vi "Cheesy_Offset.vi"(0 "Communications_Cluster":T1, 2 "Astrom_Cluster":T2 {"GuiderAstrom"."CRVAL" format="%.6g"; "GuiderAstrom"."CD" format="%_7g"; "FieldAstrom"."CRVAL" format="%.6g"; "FieldAstrom"."CD" format="%_7g"; "TablesAstrom"."CRVAL" format="%.6g"; "TablesAstrom"."CD" format="%_7g"}, 5 "RA offset":dbl format="%.2f", 9 "DEC offset":dbl format="%.2f", 11 "VariablesReferences":T3, 13 "OffsetAccuracy (pixels)":dbl=3.0) -> (6 "Error code":u8, 8 "Undo offset":bool, 10 "Warning code":u8, 15 "Error Comment":string)   [LabVIEW 2019]
uses:
  Polymorphics/Distance(single).vi
  Globals.vi
panel:
  in  "MainTAB":enum32{"Entrées", "Locales", "Sories"}(tab)
  in  "USNO_data":string[][](array[string])
  in  "FOV":dbl format="%.2f"
  in  "EPOCH":dbl format="%.2f"
  out "LimXPesto":refnum<vi>
  out "BrasPesto":refnum<vi>
  out "SNR":refnum<vi>
  out "RA before":dbl
  out "DEC before":dbl
  out "StopServo":refnum<vi>
  out "TCS VRN":refnum<visa-resource-name>
  out "Table VRN":refnum<visa-resource-name>
  out "TCS Error":errorcluster
  out "Table Error":errorcluster
  out "FieldAstrom":T4 {"CRVAL" format="%.6g"; "CD" format="%_7g"}
  out "GuiderAstrom":T4 {"CRVAL" format="%.6g"; "CD" format="%_7g"}
  out "TablesAstrom":T4 {"CRVAL" format="%.6g"; "CD" format="%_7g"}
  out "TCS Actif":refnum<vi>
  out "Table Actif":refnum<vi>
  out "StartServo":refnum<vi>
  out "Undo startguide":bool
  out "Guiding":bool caption="Guider was running"
  out "Accesible?":bool
  out "New Source Found ?":bool
  out "RA Moffset":dbl format="%.2f"
  out "DEC Moffset":dbl format="%.2f"
  out "RA Goffset":dbl=10.0 format="%.2f"
  out "DEC Goffset":dbl=10.0 format="%.2f"
  out "Goffset":bool
  out "Moffset":bool
  out "RA after":dbl
  out "DEC after":dbl
  out "cible Y":dbl
  out "cible X":dbl
  out "Servo":refnum<vi>
  out "GuiderMode":u16
  out "Mode":refnum<vi>
  out "FoyerSonde":refnum<vi>
  out "Diff X":refnum<vi>
  out "Diff Y":refnum<vi>
  out "Value X":dbl
  out "Value Y":dbl
  out "TabMove":refnum<vi>
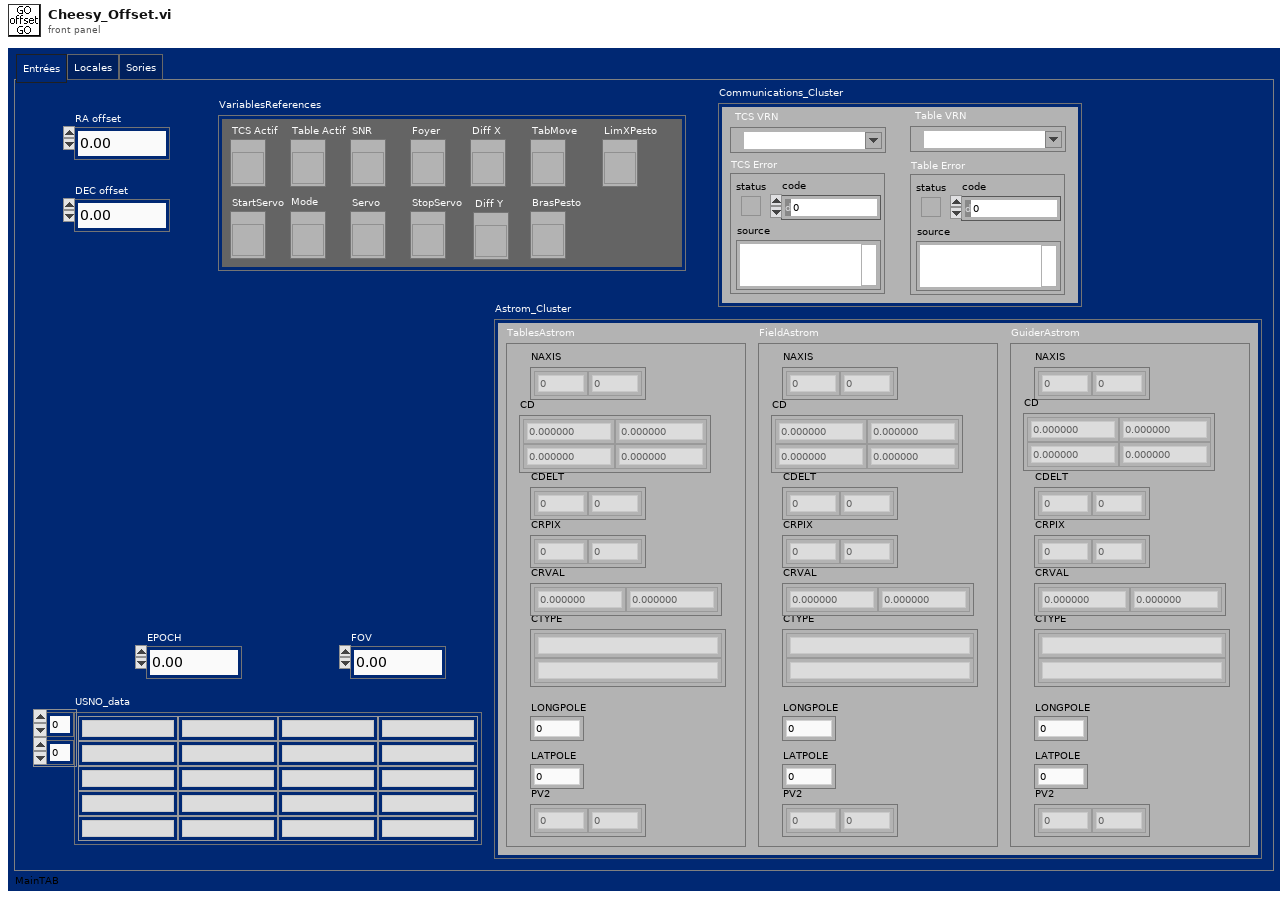
[diagram p1: front panel]
types:
  T1 = cluster{"TCS VRN":refnum<visa-resource-name>, "TCS Error":errorcluster, "Table VRN":refnum<visa-resource-name>, "Table Error":errorcluster}
  T2 = cluster{"TablesAstrom":cluster{"NAXIS":dbl[], "CD":dbl[][], "CDELT":dbl[], "CRPIX":dbl[], "CTYPE":string[], "CRVAL":dbl[], "LONGPOLE":dbl, "LATPOLE":dbl, "PV2":dbl[]}, "FieldAstrom":cluster{"NAXIS":dbl[], "CD":dbl[][], "CDELT":dbl[], "CRPIX":dbl[], "CTYPE":string[], "CRVAL":dbl[], "LONGPOLE":dbl, "LATPOLE":dbl, "PV2":dbl[]}, "GuiderAstrom":cluster{"NAXIS":dbl[], "CD":dbl[][], "CDELT":dbl[], "CRPIX":dbl[], "CTYPE":string[], "CRVAL":dbl[], "LONGPOLE":dbl, "LATPOLE":dbl, "PV2":dbl[]}}
  T3 = cluster{"TCS Actif":refnum<vi>, "Table Actif":refnum<vi>, "Foyer":refnum<vi>, "StartServo":refnum<vi>, "Mode":refnum<vi>, "Servo":refnum<vi>, "StopServo":refnum<vi>, "Diff X":refnum<vi>, "Diff Y":refnum<vi>, "SNR":refnum<vi>, "TabMove":refnum<vi>, "BrasPesto":refnum<vi>, "LimXPesto":refnum<vi>}
  T4 = cluster{"NAXIS":dbl[], "CD":dbl[][], "CDELT":dbl[], "CRPIX":dbl[], "CTYPE":string[], "CRVAL":dbl[], "LONGPOLE":dbl, "LATPOLE":dbl, "PV2":dbl[]}
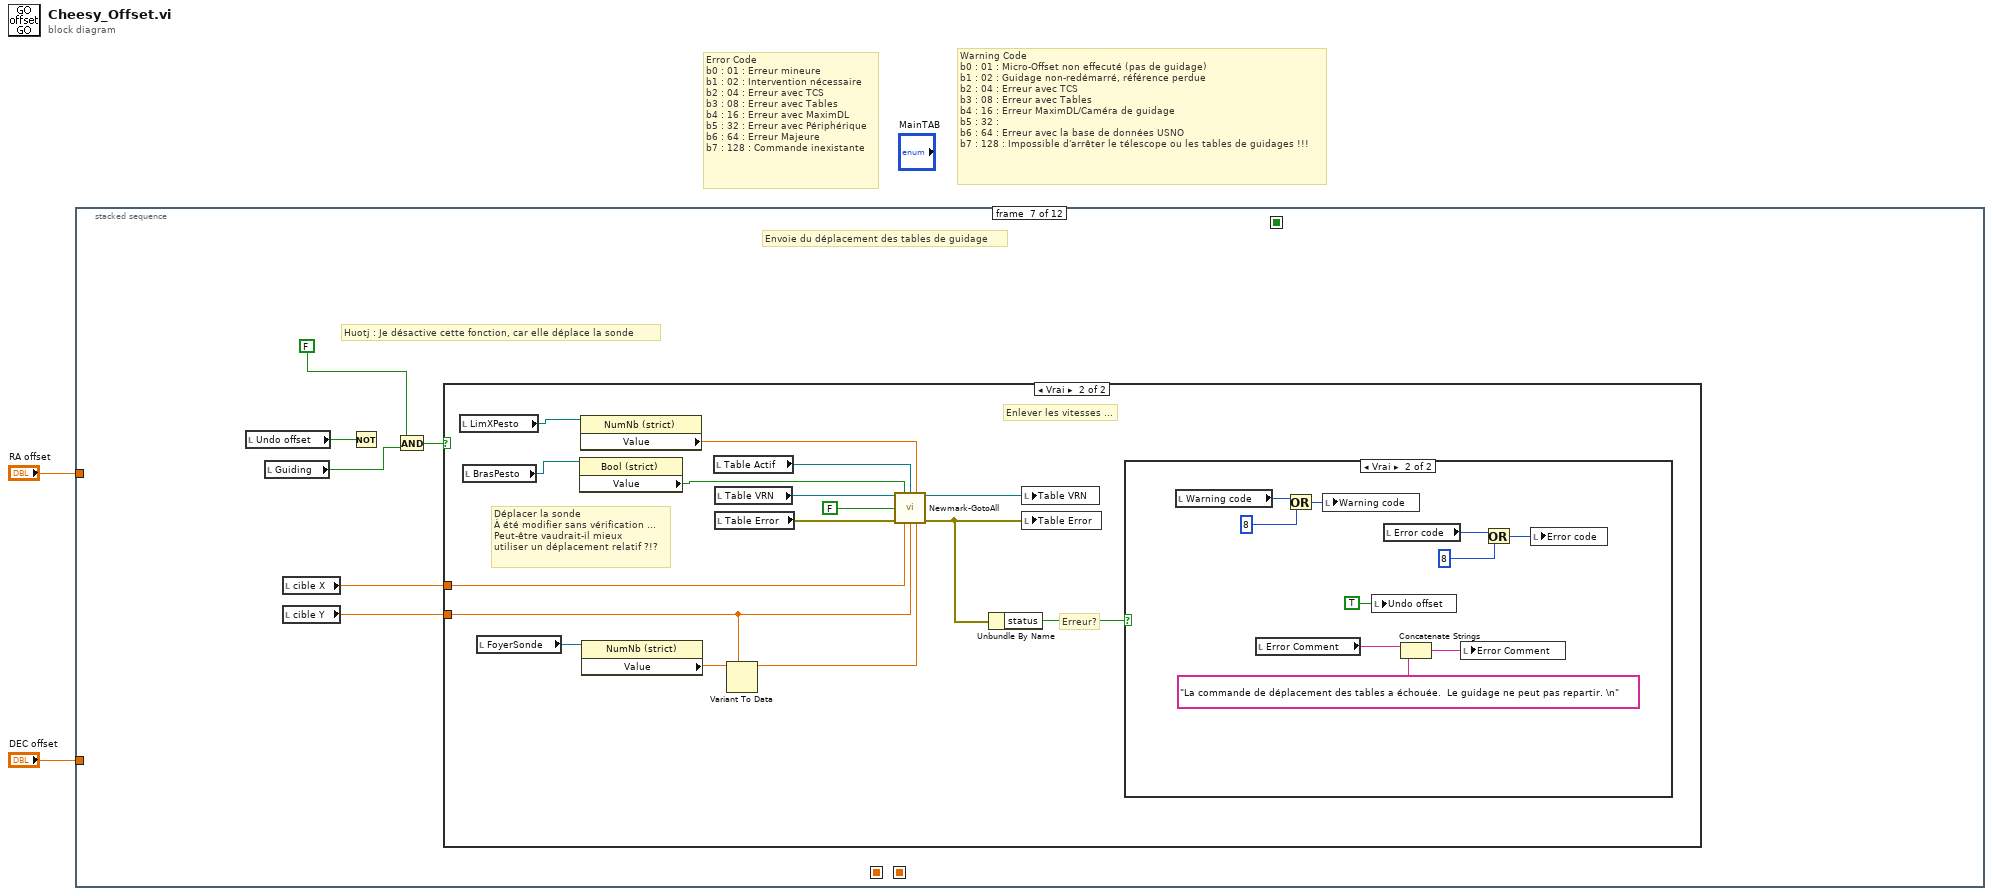
[diagram p0: block diagram]
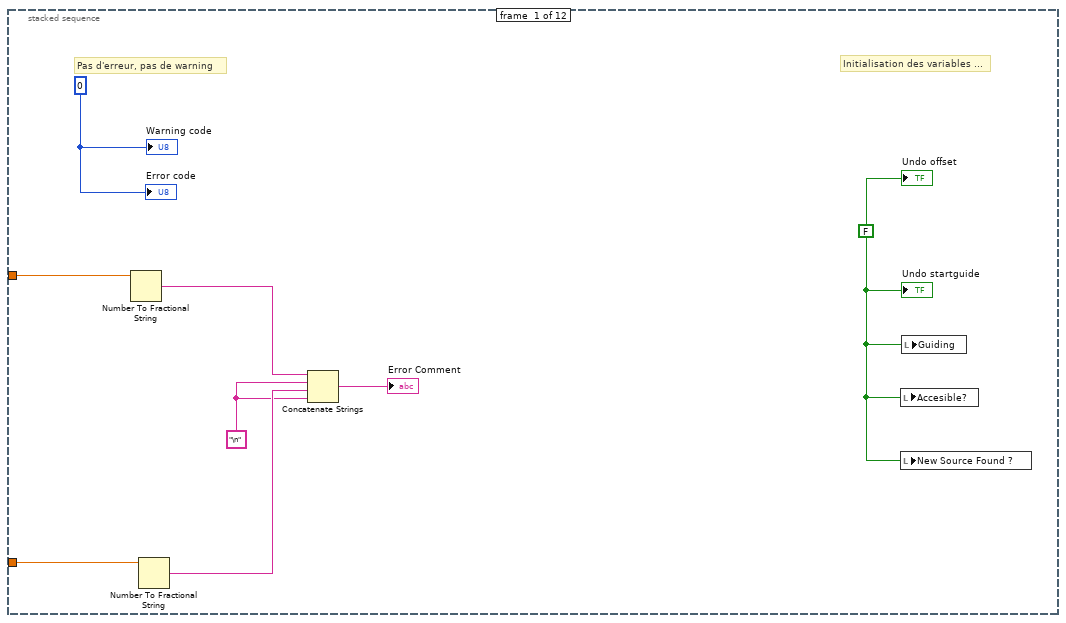
[diagram p2: hidden frame]
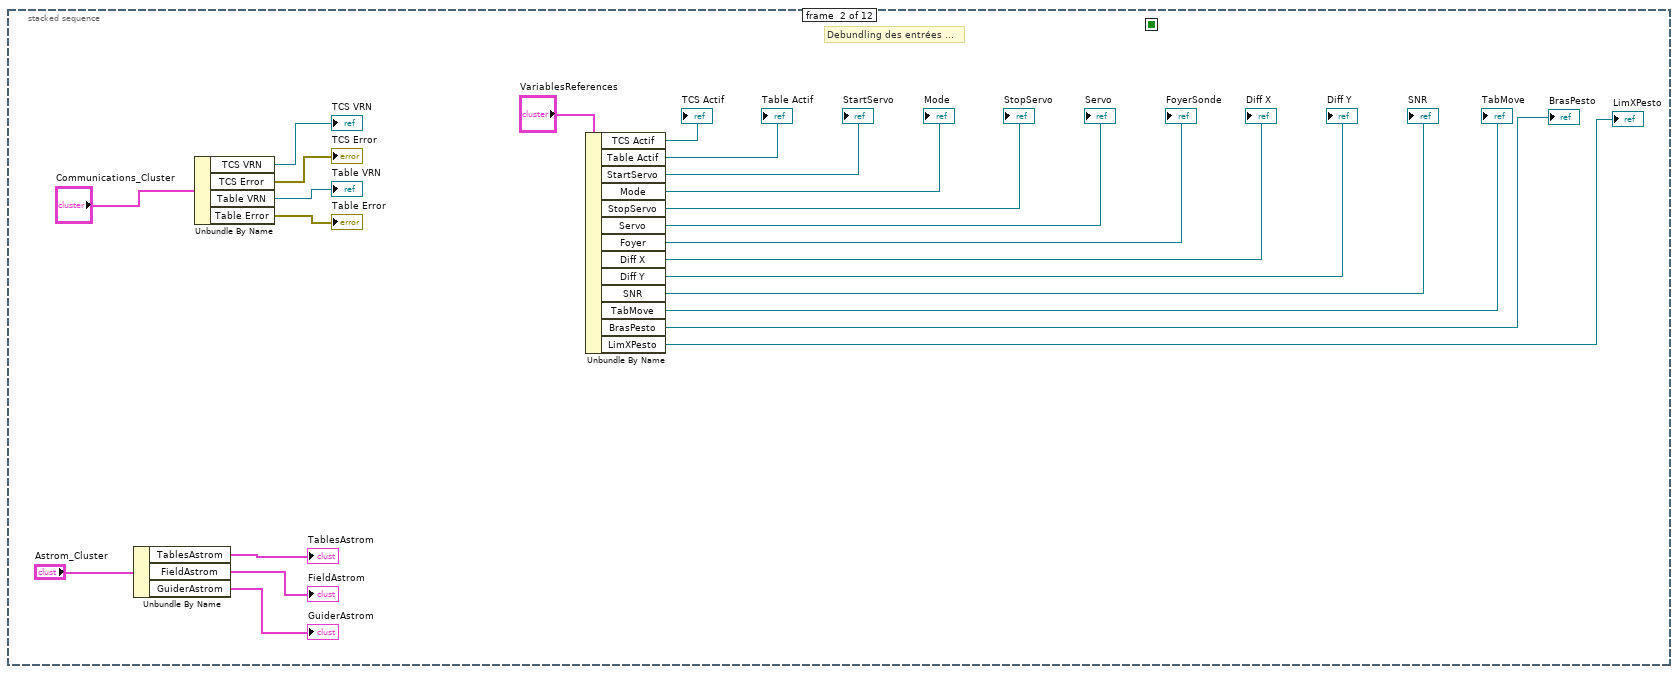
[diagram p3: hidden frame]
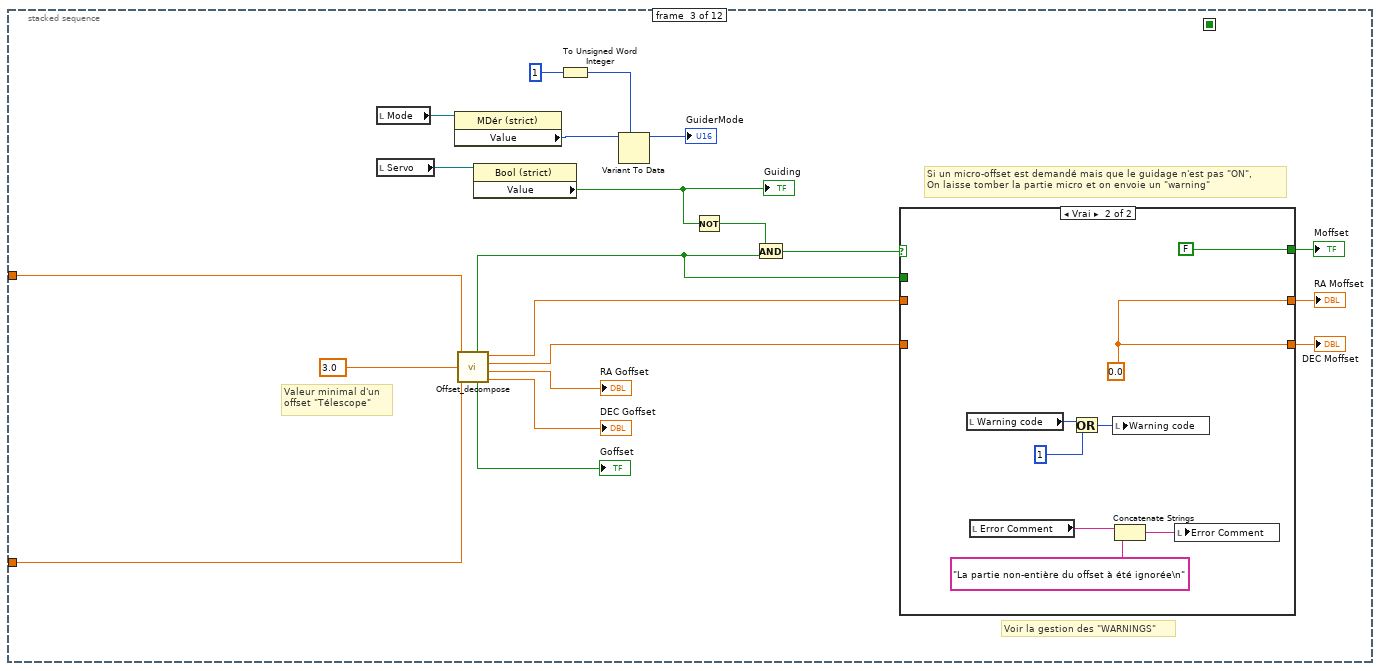
[diagram p4: hidden frame]
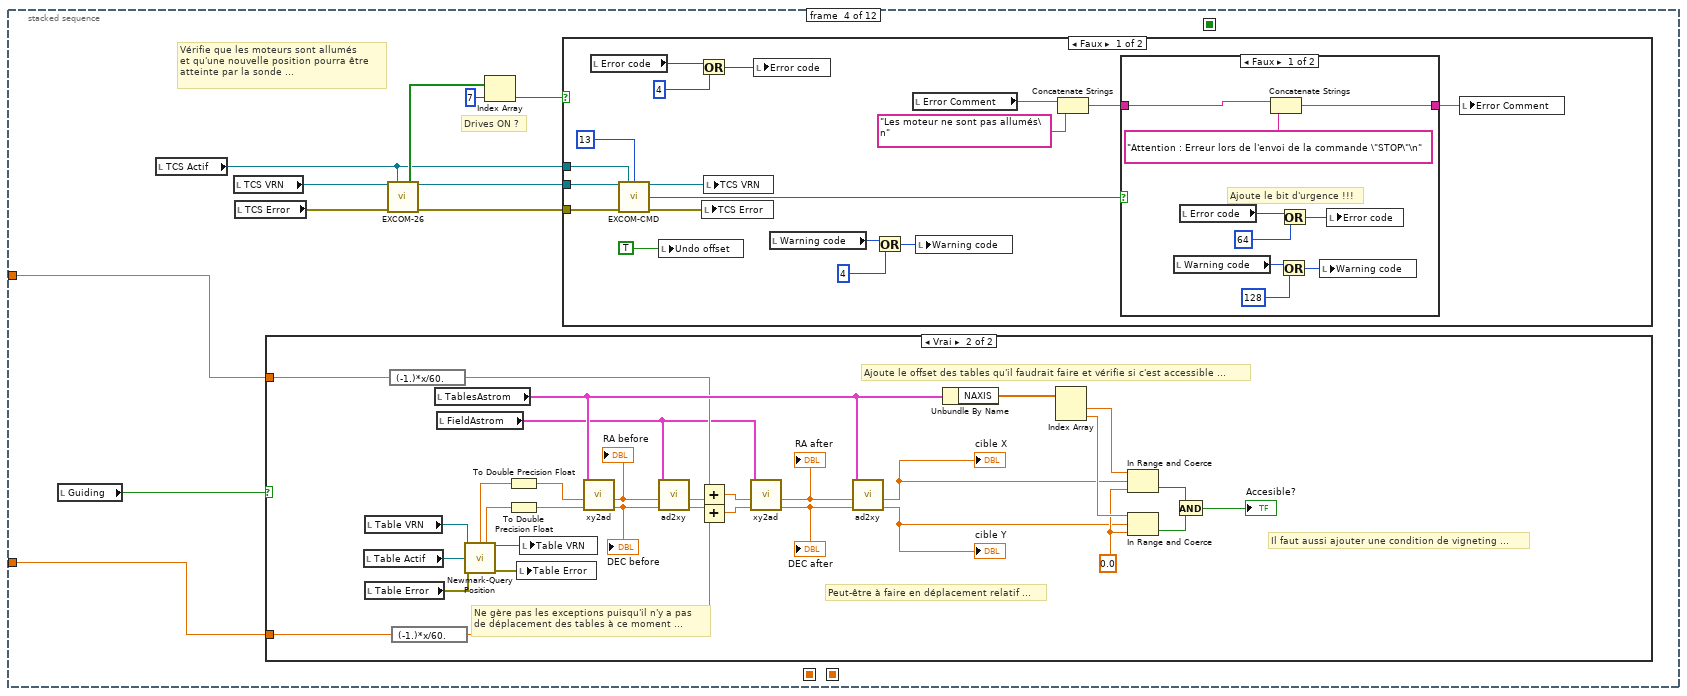
[diagram p6: hidden frame]
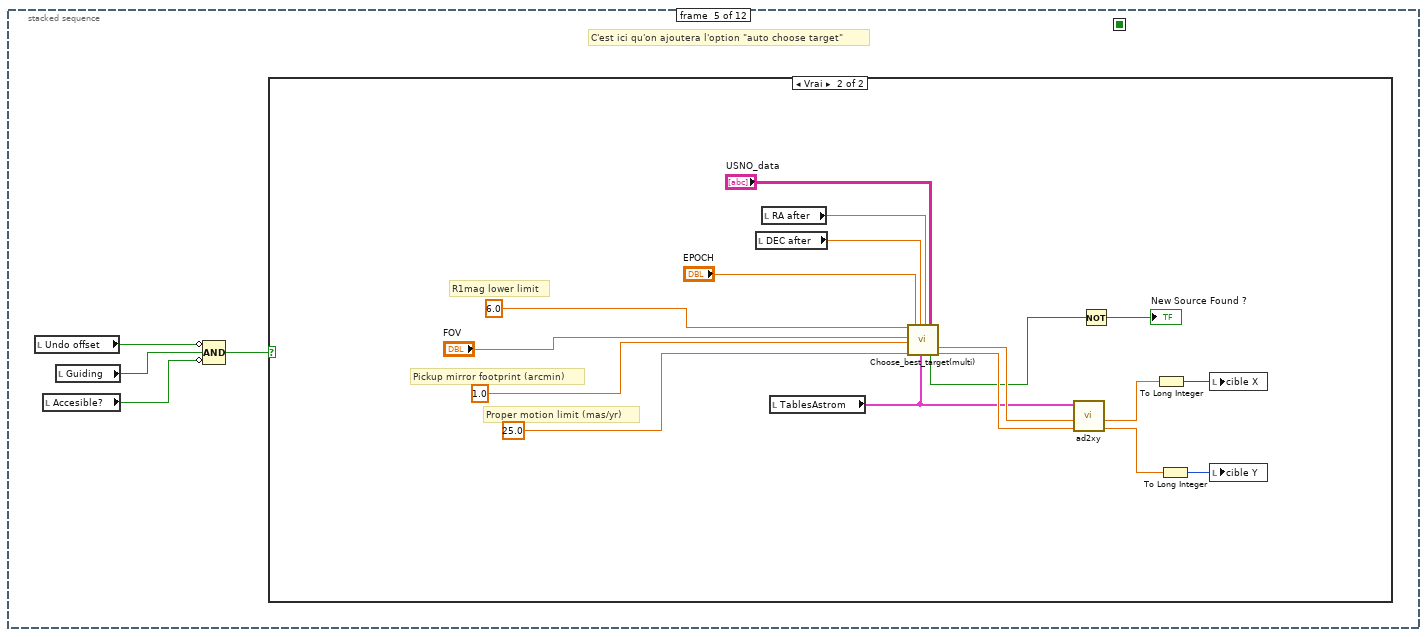
[diagram p10: hidden frame]
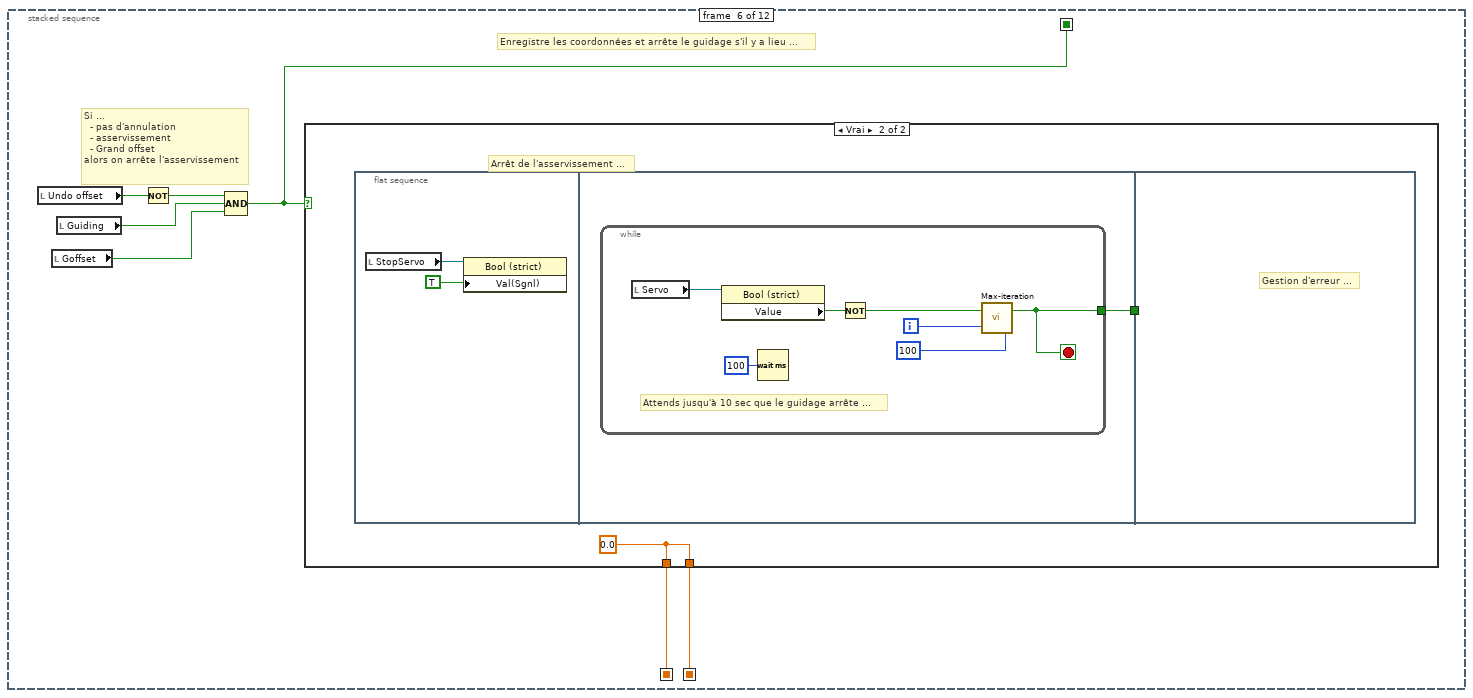
[diagram p12: hidden frame]
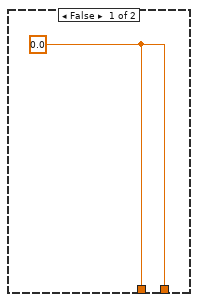
[diagram p13: hidden frame]
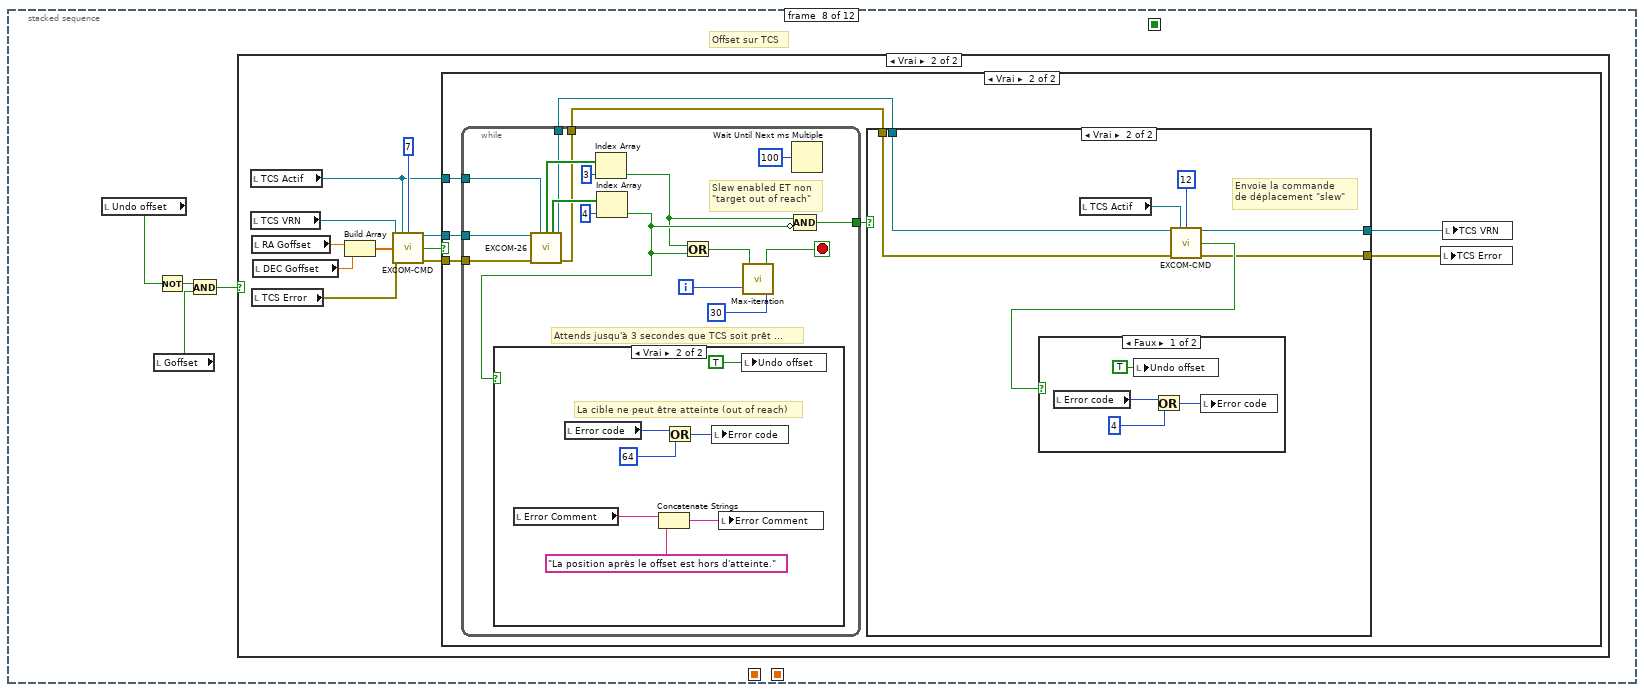
[diagram p16: hidden frame]
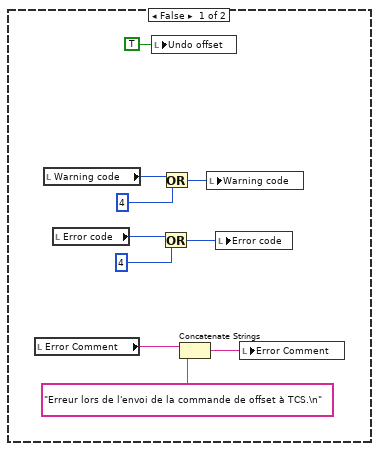
[diagram p18: hidden frame]
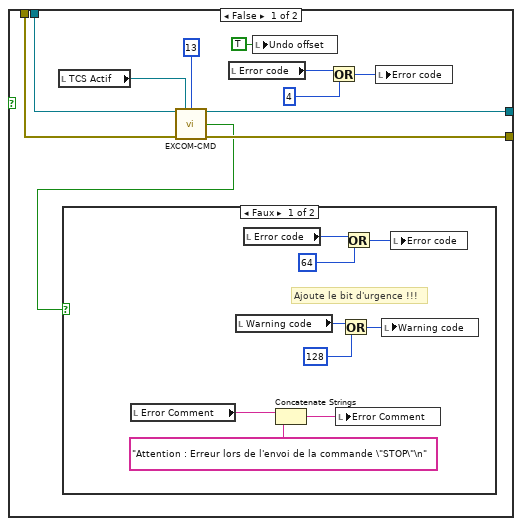
[diagram p20: hidden frame]
diagram:
  # "Error Code\nb0 : 01 : Erreur mineure\nb1 : 02 : Intervention nécessaire\nb2 : 04 : Erreur avec TCS\nb3 : 08 : Erreur avec Tables\nb4 : 16 : Erreur avec MaximDL\nb5 : 32 : Erreur avec Périphérique\nb6 : 64 : Erreur Majeure\nb7 : 128 : Commande inexistante"
  # "Warning Code\nb0 : 01 : Micro-Offset non effecuté (pas de guidage)\nb1 : 02 : Guidage non-redémarré, référence perdue\nb2 : 04 : Erreur avec TCS\nb3 : 08 : Erreur avec Tables\nb4 : 16 : Erreur MaximDL/Caméra de guidage\nb5 : 32 : \nb6 : 64 : Erreur avec la base de données USNO\nb7 : 128 : Impossible d'arrêter le télescope ou les tables de guidages !!!"
  n1 = stacked-sequence {
    seq-local: [_ _ _ _ _ w161 _ _ _ _ _ _] -> [_ _ _ _ _ _ _ _ _ _ _ _]
    seq-local: [_ _ _ _ _ w160 _ _ _ _ _ _] -> [_ _ _ _ _ _ _ _ _ _ _ _]
    seq-local: [_ _ _ _ _ w159 _ _ _ _ _ _] -> [_ _ _ _ _ _ _ _ _ _ _ _]
    tunnel: "DEC offset" -> [w7 _ w53 w74 _ _ _ _ _ _ _ _]
    tunnel: "RA offset" -> [w8 _ w54 w73 _ _ _ _ _ _ _ _]
    frame #0 {
      w3 = "\n"
      w9 = FALSE
      w10 = u8 0
      # "Initialisation des variables ..."
      # "Pas d'erreur, pas de warning"
      n2 = Number To Fractional String(number=w8) -> (F-format string=w6:string)  [unwired: 3 in]
      n3 = Number To Fractional String(number=w7) -> (F-format string=w5:string)  [unwired: 3 in]
      n4 = Concatenate Strings(w6, w3, w5, w3) -> (→"Error Comment":string)
      n5 = local write "Accesible?"(w9) -> ()
      n6 = local write "New Source Found ?"(w9) -> ()
      n7 = local write "Guiding"(w9) -> ()
      "Error code" <- w10
      "Warning code" <- w10
      "Undo offset" <- w9
      "Undo startguide" <- w9
    }
    frame #1 {
      # "Debundling des entrées ..."
      n8 = Unbundle By Name("Astrom_Cluster") -> ("TablesAstrom"=→"TablesAstrom":T4, "FieldAstrom"=→"FieldAstrom":T4, "GuiderAstrom"=→"GuiderAstrom":T4)
      n9 = Unbundle By Name("Communications_Cluster") -> ("TCS VRN"=→"TCS VRN":refnum<visa-resource-name>, "TCS Error"=→"TCS Error":errorcluster, "Table VRN"=→"Table VRN":refnum<visa-resource-name>, "Table Error"=→"Table Error":errorcluster)
      n10 = Unbundle By Name("VariablesReferences") -> ("TCS Actif"=→"TCS Actif":refnum<vi>, "Table Actif"=→"Table Actif":refnum<vi>, "StartServo"=→"StartServo":refnum<vi>, "Mode"=→"Mode":refnum<vi>, "StopServo"=→"StopServo":refnum<vi>, "Servo"=→"Servo":refnum<vi>, "Foyer"=→"FoyerSonde":refnum<vi>, "Diff X"=→"Diff X":refnum<vi>, "Diff Y"=→"Diff Y":refnum<vi>, "SNR"=→"SNR":refnum<vi>, "TabMove"=→"TabMove":refnum<vi>, "BrasPesto"=→"BrasPesto":refnum<vi>, "LimXPesto"=→"LimXPesto":refnum<vi>)
    }
    frame #2 {
      # "Voir la gestion des \"WARNINGS\""
      # "Si un micro-offset est demandé mais que le guidage n'est pas \"ON\",\nOn laisse tomber la partie micro et on envoie un \"warning\""
      # "Valeur minimal d'un\noffset \"Télescope\""
      n11 = local read "Mode"() -> (w34:refnum<vi>)
      n12 = local read "Servo"() -> (w40:refnum<vi>)
      n13 = property class="MDér (strict)"(reference=w34) -> ("Value"=w38:u16)  [unwired: 1 in, 2 out]
      n14 = call "Offset_decompose.vi"("DEC offset"=w53, "RA offset"=w54, "Micro Limit"=3.0 ("y")) -> ("Goffset"=→"Goffset":bool, "Moffset"=w43:bool, "DEC Goffset"=→"DEC Goffset":dbl, "RA Goffset"=→"RA Goffset":dbl, "DEC Moffset"=w47:dbl, "RA Moffset"=w48:dbl)  [unwired: 2 in]
      n15 = property class="Bool (strict)"(reference=w40) -> ("Value"=w39:bool)  [unwired: 1 in, 2 out]
      "Guiding" <- w39
      n16 = To Unsigned Word Integer(number=u8 1) -> (unsigned 16bit integer=w36:u16)
      n17 = Variant To Data(type=w36, Variant=w38) -> (data=→"GuiderMode":u16)  [unwired: 1 in, 1 out]
      n18 = Not(x=w39) -> (.not. x?=w49:bool)
      n19 = And(x=w49, y=w43) -> (x .and. y?=w44:bool)
      n20 = case shown="Vrai" w44 {
        tunnel: w48 -> [w57 _]
        tunnel: w47 -> [w56 _]
        tunnel: [w57 w64] -> w46
        tunnel: [w56 w64] -> w45
        tunnel: w43 -> [w55 _]
        tunnel: [w55 FALSE] -> w41
        frame False {
        }
        frame True {
          w64 = 0.0
          n21 = local read "Warning code"() -> (w63:u8)
          n22 = local read "Error Comment"() -> (w60:string)
          n23 = Or(x=w63, y=u8 1) -> (x .or. y?=w62:u8)
          n24 = local write "Warning code"(w62) -> ()
          n25 = Concatenate Strings(w60, "La partie non-entière du offset à été ignorée\n") -> (w59:string)
          n26 = local write "Error Comment"(w59) -> ()
        }
      }
      "DEC Moffset" <- w45
      "RA Moffset" <- w46
      "Moffset" <- w41
    }
    frame #3 {
      # "Drives ON ?"
      # "Vérifie que les moteurs sont allumés\net qu'une nouvelle position pourra être\natteinte par la sonde ..."
      n27 = local read "Guiding"() -> (w72:bool)
      n28 = local read "TCS Actif"() -> (w68:refnum<vi>)
      n29 = local read "TCS VRN"() -> (w67:refnum<visa-resource-name>)
      n30 = local read "TCS Error"() -> (w66:errorcluster)
      n31 = case shown="Vrai" w72 {
        tunnel: w74 -> [_ w106]
        tunnel: w73 -> [_ w105]
        frame False {
        }
        frame True {
          w98 = 0.0
          # "Peut-être à faire en déplacement relatif ..."
          # "Ne gère pas les exceptions puisqu'il n'y a pas\nde déplacement des tables à ce moment ..."
          # "Il faut aussi ajouter une condition de vigneting ..."
          # "Ajoute le offset des tables qu'il faudrait faire et vérifie si c'est accessible ..."
          n32 = local read "Table Actif"() -> (w84:refnum<vi>)
          n33 = local read "Table VRN"() -> (w82:refnum<visa-resource-name>)
          n34 = local read "Table Error"() -> (w80:errorcluster)
          n35 = expression code="(-1.)*x/60."(w105) -> (w94:dbl)
          n36 = expression code="(-1.)*x/60."(w106) -> (w93:dbl)
          n37 = local read "TablesAstrom"() -> (w104:T4)
          n38 = local read "FieldAstrom"() -> (w83:T4)
          n39 = call "Newmark-QueryPosition.vi"("Table VRN IN"=w82, "Bool Refnum"=w84, "Error IN"=w80) -> ("X Axis"=w86:dbl, "Y Axis"=w85:dbl, "Table VRN OUT"=w79:refnum<visa-resource-name>, "Error OUT"=w81:errorcluster)  [unwired: 5 in, 4 out]
          n40 = To Double Precision Float(number=w86) -> (double precision float=w108:dbl)
          n41 = To Double Precision Float(number=w85) -> (double precision float=w107:dbl)
          n42 = local write "Table Error"(w81) -> ()
          n43 = local write "Table VRN"(w79) -> ()
          n44 = call "xy2ad.vi"("Y (px)"=w107, "X (px)"=w108, "Astrometry"=w104) -> ("DEC (°)"=w77:dbl, "RA (°)"=w78:dbl)  [unwired: 5 in, 2 out]
          "RA before" <- w78
          "DEC before" <- w77
          n45 = call "ad2xy.vi"("DEC"=w77, "RA"=w78, "Astrometry"=w83) -> ("Y"=w95:dbl, "X"=w96:dbl)  [unwired: 6 in, 1 out]
          n46 = Add(x=w94, y=w96) -> (x+y=w92:dbl)
          n47 = Add(x=w95, y=w93) -> (x+y=w91:dbl)
          n48 = call "xy2ad.vi"("Y (px)"=w91, "X (px)"=w92, "Astrometry"=w83) -> ("DEC (°)"=w89:dbl, "RA (°)"=w90:dbl)  [unwired: 5 in, 2 out]
          "DEC after" <- w89
          "RA after" <- w90
          n49 = call "ad2xy.vi"("DEC"=w89, "RA"=w90, "Astrometry"=w104) -> ("Y"=w87:dbl, "X"=w88:dbl)  [unwired: 6 in, 1 out]
          "cible X" <- w88
          "cible Y" <- w87
          n50 = Unbundle By Name(w104) -> ("NAXIS"=w103:dbl[])
          n51 = Index Array(array=w103) -> (element #1=w102:dbl, element #2=w101:dbl)  [unwired: 2 in]
          n52 = In Range and Coerce(upper limit=w102, x=w88, lower limit=w98) -> (In Range?=w100:bool)  [unwired: 1 out]
          n53 = In Range and Coerce(upper limit=w101, x=w87, lower limit=w98) -> (In Range?=w99:bool)  [unwired: 1 out]
          n54 = And(x=w100, y=w99) -> (x .and. y?=→"Accesible?":bool)
        }
      }
      n55 = call "EXCOM-26.vi"("VRN IN"=w67, "Bool Refnum"=w68, "Error IN"=w66) -> ("STATH"=w70:bool[], "VRN OUT"=w75:refnum<visa-resource-name>, "Error OUT"=w69:errorcluster)  [unwired: 6 in, 4 out]
      n56 = Index Array(array=w70, index=7 ("Index")) -> (element=w76:bool)
      n57 = case shown="Faux" w76 {
        tunnel: w75 -> [w121 _]
        tunnel: w69 -> [w116 _]
        tunnel: w68 -> [w115 _]
        frame False {
          n58 = local read "Error code"() -> (w126:u8)
          n59 = call "EXCOM-CMD.vi"("VRN IN"=w121, "Bool Refnum"=w115, "Commande #"=13 ("NombredArguments"), "Error IN"=w116) -> ("VRN OUT"=w110:refnum<visa-resource-name>, "OK Done"=w122:bool, "Error OUT"=w109:errorcluster)  [unwired: 9 in]
          n60 = local write "Undo offset"(TRUE) -> ()
          n61 = Or(x=w126, y=u8 4) -> (x .or. y?=w125:u8)
          n62 = local write "TCS Error"(w109) -> ()
          n63 = local write "TCS VRN"(w110) -> ()
          n64 = local write "Error code"(w125) -> ()
          n65 = local read "Warning code"() -> (w120:u8)
          n66 = Or(x=w120, y=u8 4) -> (x .or. y?=w119:u8)
          n67 = local read "Error Comment"() -> (w114:string)
          n68 = local write "Warning code"(w119) -> ()
          n69 = Concatenate Strings(w114, "Les moteur ne sont pas allumés\n") -> (w112:string)
          n70 = case shown="Faux" w122 {
            tunnel: w112 -> [w129 w136]
            tunnel: [w128 w136] -> w111
            frame False {
              # "Ajoute le bit d'urgence !!!"
              n71 = local read "Warning code"() -> (w133:u8)
              n72 = local read "Error code"() -> (w132:u8)
              n73 = Concatenate Strings(w129, "Attention : Erreur lors de l'envoi de la commande \"STOP\"\n" ("string")) -> (w128:string)
              n74 = Or(x=w133, y=u8 128) -> (x .or. y?=w134:u8)
              n75 = Or(x=w132, y=u8 64) -> (x .or. y?=w131:u8)
              n76 = local write "Warning code"(w134) -> ()
              n77 = local write "Error code"(w131) -> ()
            }
            frame True {
            }
          }
          n78 = local write "Error Comment"(w111) -> ()
        }
        frame True {
        }
      }
    }
    frame #4 {
      # "C'est ici qu'on ajoutera l'option \"auto choose target\""
      n79 = local read "Undo offset"() -> (w140:bool)
      n80 = local read "Accesible?"() -> (w138:bool)
      n81 = local read "Guiding"() -> (w139:bool)
      n82 = Compound Arithmetic op=AND(invert w140, w139, invert w138) -> (w137:bool)
      n83 = case shown="Vrai" w137 {
        frame False {
        }
        frame True {
          # "Proper motion limit (mas/yr)"
          # "Pickup mirror footprint (arcmin)"
          # "R1mag lower limit"
          n84 = local read "DEC after"() -> (w156:dbl)
          n85 = local read "RA after"() -> (w157:dbl)
          n86 = local read "TablesAstrom"() -> (w147:T4)
          n87 = call "Choose_best_target(multi).vi"("R1mag lower limit"=6.0, "FOV"="FOV", "Footprint"=1.0, "PM limit"=25.0 ("Footprint"), "EPOCH TEL"="EPOCH", "DEC TEL"=w156, "Table Astrometry"=w147, "RA TEL"=w157, "USNO_data"="USNO_data") -> ("erreur"=w142:bool, "target RA (deg)"=w150:dbl, "target DEC (deg)"=w149:dbl)  [unwired: 3 in, 5 out]
          n88 = call "ad2xy.vi"("DEC"=w149, "RA"=w150, "Astrometry"=w147) -> ("Y"=w151:dbl, "X"=w152:dbl)  [unwired: 6 in, 1 out]
          n89 = Not(x=w142) -> (.not. x?=→"New Source Found ?":bool)
          n90 = To Long Integer(number=w152) -> (32bit integer=w154:i32)
          n91 = To Long Integer(number=w151) -> (32bit integer=w153:i32)
          n92 = local write "cible X"(w154) -> ()
          n93 = local write "cible Y"(w153) -> ()
        }
      }
    }
    frame #5 {
      # "Si ...\n  - pas d'annulation\n  - asservissement\n  - Grand offset\nalors on arrête l'asservissement"
      # "Enregistre les coordonnées et arrête le guidage s'il y a lieu ..."
      n94 = local read "Undo offset"() -> (w163:bool)
      n95 = local read "Goffset"() -> (w158:bool)
      n96 = local read "Guiding"() -> (w162:bool)
      n97 = Not(x=w163) -> (.not. x?=w164:bool)
      n98 = Compound Arithmetic op=AND(w164, w162, w158) -> (w161:bool)
      n99 = case shown="Vrai" w161 {
        tunnel: [w165 w167] -> w159
        tunnel: [w165 w167] -> w160
        frame False {
          w165 = sgl 0.0 ("GuiderYError")
        }
        frame True {
          w167 = sgl 0.0 ("GuiderYError")
          # "Arrêt de l'asservissement ..."
          n100 = flat-sequence {
            tunnel: [w170] -> w166
            tunnel: w166 -> [_]
            frame #0 {
              n101 = local read "StopServo"() -> (w169:refnum<vi>)
              n102 = property class="Bool (strict)"(reference=w169, "Val(Sgnl)"=TRUE ("Value (Signaling)")) -> ()  [unwired: 1 in, 2 out]
            }
            frame #1 {
              n103 = while {
                tunnel: [w172] -> w170
                i -> [w175]
                stop <- w172 stop-if-true
                # "Attends jusqu'à 10 sec que le guidage arrête ..."
                n104 = local read "Servo"() -> (w177:refnum<vi>)
                n105 = property class="Bool (strict)"(reference=w177) -> ("Value"=w176:bool)  [unwired: 1 in, 2 out]
                n106 = Wait (ms)(milliseconds to wait=u32 100) -> ()  [unwired: 1 out]
                n107 = Not(x=w176) -> (.not. x?=w171:bool)
                n108 = call "Max-iteration.vi"("i max"=100, "i act"=w175, "Valeur entrante"=w171) -> ("break ?"=w172:bool)
              }
            }
            frame #2 {
              # "Gestion d'erreur ..."
            }
          }
        }
      }
    }
    frame #6 {
      # "Huotj : Je désactive cette fonction, car elle déplace la sonde"
      # "Envoie du déplacement des tables de guidage"
      n109 = local read "Undo offset"() -> (w180:bool)
      n110 = local read "Guiding"() -> (w179:bool)
      n111 = local read "cible X"() -> (w183:dbl)
      n112 = local read "cible Y"() -> (w182:dbl)
      n113 = Not(x=w180) -> ()  [unwired: 1 out]
      n114 = And(x=FALSE, y=w179) -> (x .and. y?=w181:bool)
      n115 = case shown="Vrai" w181 {
        tunnel: w182 -> [_ w189]
        tunnel: w183 -> [_ w198]
        frame False {
        }
        frame True {
          # "Erreur?"
          # "Enlever les vitesses ..."
          # "Déplacer la sonde\nÀ été modifier sans vérification ...\nPeut-être vaudrait-il mieux\nutiliser un déplacement relatif ?!?"
          n116 = local read "LimXPesto"() -> (w187:refnum<vi>)
          n117 = local read "BrasPesto"() -> (w185:refnum<vi>)
          n118 = local read "FoyerSonde"() -> (w191:refnum<vi>)
          n119 = property class="Bool (strict)"(reference=w185) -> ("Value"=w184:bool)  [unwired: 1 in, 2 out]
          n120 = property on="Property Node" class="NumNb (strict)"(reference=w187) -> ("Value"=w186:dbl)  [unwired: 1 in, 2 out]
          n121 = property on="Property Node" class="NumNb (strict)"(reference=w191) -> ("Value"=w190:dbl)  [unwired: 1 in, 2 out]
          n122 = local read "Table Actif"() -> (w195:refnum<vi>)
          n123 = local read "Table VRN"() -> (w193:refnum<visa-resource-name>)
          n124 = local read "Table Error"() -> (w194:errorcluster)
          n125 = Variant To Data(type=w189, Variant=w190) -> (data=w188:dbl)  [unwired: 1 in, 1 out]
          n126 = call "Newmark-GotoAll.vi"("Table VRN IN"=w193, "BrasPesto"=w184, "Bool Refnum"=w195, "LimXPesto"=w186, "Notify?"=FALSE, "Error IN"=w194, "Position X"=w198, "Position Y"=w189, "Position Z"=w188) -> ("Table VRN OUT"=w196:refnum<visa-resource-name>, "Error OUT"=w197:errorcluster)  [unwired: 5 in]
          n127 = Unbundle By Name(w197) -> ("status"=w199:bool)
          n128 = local write "Table VRN"(w196) -> ()
          n129 = local write "Table Error"(w197) -> ()
          n130 = case shown="Vrai" w199 {
            frame False {
            }
            frame True {
              n131 = local read "Warning code"() -> (w205:u8)
              n132 = local read "Error Comment"() -> (w202:string)
              n133 = Or(x=w205, y=u8 8) -> (x .or. y?=w204:u8)
              n134 = local write "Warning code"(w204) -> ()
              n135 = local write "Undo offset"(TRUE) -> ()
              n136 = local read "Error code"() -> (w206:u8)
              n137 = Concatenate Strings(w202, "La commande de déplacement des tables a échouée.  Le guidage ne peut pas repartir. \n") -> (w201:string)
              n138 = local write "Error Comment"(w201) -> ()
              n139 = Or(x=w206, y=u8 8) -> (x .or. y?=w207:u8)
              n140 = local write "Error code"(w207) -> ()
            }
          }
        }
      }
    }
    frame #7 {
      # "Offset sur TCS"
      n141 = local read "Undo offset"() -> (w211:bool)
      n142 = local read "Goffset"() -> (w210:bool)
      n143 = Not(x=w211) -> (.not. x?=w212:bool)
      n144 = And(x=w212, y=w210) -> (x .and. y?=w213:bool)
      n145 = case shown="Vrai" w213 {
        frame False {
        }
        frame True {
          n146 = local read "TCS Actif"() -> (w216:refnum<vi>)
          n147 = local read "TCS VRN"() -> (w214:refnum<visa-resource-name>)
          n148 = local read "RA Goffset"() -> (w218:dbl)
          n149 = local read "TCS Error"() -> (w215:errorcluster)
          n150 = local read "DEC Goffset"() -> (w219:dbl)
          n151 = Build Array(w218, w219) -> (w217:dbl[])
          n152 = call "EXCOM-CMD.vi"("VRN IN"=w214, "Bool Refnum"=w216, "Commande #"=7 ("NombredArguments"), "Args"=w217, "Error IN"=w215) -> ("VRN OUT"=w222:refnum<visa-resource-name>, "OK Done"=w223:bool, "Error OUT"=w220:errorcluster)  [unwired: 8 in]
          n153 = case shown="Vrai" w223 {
            tunnel: w222 -> [_ w240]
            tunnel: w220 -> [_ w238]
            tunnel: w216 -> [_ w236]
            frame False {
              n154 = local read "Error Comment"() -> (w226:string)
              n155 = local read "Warning code"() -> (w227:u8)
              n156 = local read "Error code"() -> (w232:u8)
              n157 = local write "Undo offset"(TRUE) -> ()
              n158 = Or(x=w232, y=u8 4) -> (x .or. y?=w231:u8)
              n159 = Or(x=w227, y=u8 4) -> (x .or. y?=w228:u8)
              n160 = Concatenate Strings(w226, "Erreur lors de l'envoi de la commande de offset à TCS.\n") -> (w225:string)
              n161 = local write "Warning code"(w228) -> ()
              n162 = local write "Error code"(w231) -> ()
              n163 = local write "Error Comment"(w225) -> ()
            }
            frame True {
              n164 = while {
                tunnel: [w245] -> w241
                tunnel: w240 -> [w253]
                tunnel: [w252] -> w239
                tunnel: w238 -> [w244]
                tunnel: [w243] -> w237
                tunnel: w236 -> [w242]
                i -> [w249]
                stop <- w250 stop-if-true
                # "Slew enabled ET non\n\"target out of reach\""
                # "Attends jusqu'à 3 secondes que TCS soit prêt ..."
                n165 = call "EXCOM-26.vi"("VRN IN"=w253, "Bool Refnum"=w242, "Error IN"=w244) -> ("STATL"=w255:bool[], "STATH"=w254:bool[], "VRN OUT"=w252:refnum<visa-resource-name>, "Error OUT"=w243:errorcluster)  [unwired: 6 in, 3 out]
                n166 = Index Array(array=w255, index=3 ("Index")) -> (element=w246:bool)
                n167 = Index Array(array=w254, index=4 ("Index")) -> (element=w247:bool)
                n168 = case shown="Vrai" w247 {
                  frame False {
                  }
                  frame True {
                    # "La cible ne peut être atteinte (out of reach)"
                    n169 = local read "Error Comment"() -> (w261:string)
                    n170 = local read "Error code"() -> (w265:u8)
                    n171 = Concatenate Strings(w261, "La position après le offset est hors d'atteinte.") -> (w260:string)
                    n172 = Or(x=w265, y=u8 64) -> (x .or. y?=w264:u8)
                    n173 = local write "Error code"(w264) -> ()
                    n174 = local write "Error Comment"(w260) -> ()
                    n175 = local write "Undo offset"(TRUE ("Undo offset")) -> ()
                  }
                }
                n176 = Or(x=w246, y=w247) -> (x .or. y?=w251:bool)
                n177 = call "Max-iteration.vi"("i max"=30, "i act"=w249, "Valeur entrante"=w251) -> ("break ?"=w250:bool)
                n178 = Wait Until Next ms Multiple(millisecond multiple=u32 100 ("n millisecondes")) -> ()  [unwired: 1 out]
                n179 = Compound Arithmetic op=AND(w246, invert w247) -> (w245:bool)
              }
              n180 = case shown="Vrai" w241 {
                tunnel: w239 -> [w275 w292]
                tunnel: [w270 w289] -> w235
                tunnel: w237 -> [w269 w288]
                tunnel: [w268 w287] -> w234
                frame False {
                  n181 = local read "TCS Actif"() -> (w267:refnum<vi>)
                  n182 = call "EXCOM-CMD.vi"("VRN IN"=w275, "Bool Refnum"=w267, "Commande #"=13 ("NombredArguments"), "Error IN"=w269) -> ("VRN OUT"=w270:refnum<visa-resource-name>, "OK Done"=w266:bool, "Error OUT"=w268:errorcluster)  [unwired: 9 in]
                  n183 = case shown="Faux" w266 {
                    frame False {
                      # "Ajoute le bit d'urgence !!!"
                      n184 = local read "Error Comment"() -> (w279:string)
                      n185 = local read "Warning code"() -> (w283:u8)
                      n186 = local read "Error code"() -> (w282:u8)
                      n187 = Concatenate Strings(w279, "Attention : Erreur lors de l'envoi de la commande \"STOP\"\n" ("string")) -> (w278:string)
                      n188 = local write "Error Comment"(w278) -> ()
                      n189 = Or(x=w283, y=u8 128) -> (x .or. y?=w284:u8)
                      n190 = Or(x=w282, y=u8 64) -> (x .or. y?=w281:u8)
                      n191 = local write "Warning code"(w284) -> ()
                      n192 = local write "Error code"(w281) -> ()
                    }
                    frame True {
                    }
                  }
                  n193 = local read "Error code"() -> (w272:u8)
                  n194 = local write "Undo offset"(TRUE ("Undo offset")) -> ()
                  n195 = Or(x=w272, y=u8 4) -> (x .or. y?=w273:u8)
                  n196 = local write "Error code"(w273) -> ()
                }
                frame True {
                  # "Envoie la commande\nde déplacement \"slew\""
                  n197 = local read "TCS Actif"() -> (w286:refnum<vi>)
                  n198 = call "EXCOM-CMD.vi"("VRN IN"=w292, "Bool Refnum"=w286, "Commande #"=12, "Error IN"=w288) -> ("VRN OUT"=w289:refnum<visa-resource-name>, "OK Done"=w291:bool, "Error OUT"=w287:errorcluster)  [unwired: 9 in]
                  n199 = case shown="Faux" w291 {
                    frame False {
                      n200 = local read "Error code"() -> (w294:u8)
                      n201 = local write "Undo offset"(TRUE ("Undo offset")) -> ()
                      n202 = Or(x=w294, y=u8 4) -> (x .or. y?=w295:u8)
                      n203 = local write "Error code"(w295) -> ()
                    }
                    frame True {
                    }
                  }
                }
              }
              n204 = local write "TCS Error"(w234) -> ()
              n205 = local write "TCS VRN"(w235) -> ()
            }
          }
        }
      }
    }
    frame #8 {
      # "Attends que tous les déplacement soit complétés ..."
      n206 = local read "Undo offset"() -> (w297:bool)
      n207 = case shown="Faux" w297 {
        frame False {
          # "If NOT Monitor Table AND $\nGuiding AND NOT $\n\"Undo StartGuide\" $\nTHEN StartGuide"
          # "Ajoute les codes d'erreurs correspondants et arrête le Télescope"
          # "Attends jusqu'à 30 secondes que \"SLEW\" redevienne \"OFF\""
          # "Attends 3 sec que \"SLEW\" soit \"ON\"\nVérifier qu'il n'y a pas des cas où le\nmouvement se fait sans que le flag monte ..."
          # "Si vrai, il y a eu une erreur ..."
          n208 = local read "TCS Actif"() -> (w307:refnum<vi>)
          n209 = local read "TCS VRN"() -> (w299:refnum<visa-resource-name>)
          n210 = local read "TCS Error"() -> (w298:errorcluster)
          n211 = while {
            tunnel: [w414] -> w304
            i -> [w418]
            stop <- w417 stop-if-true
            w414 = FALSE
            # "Devra être changer quand on décidera de la\nfaçon de gérer le déplacement des tables ..."
            # "Attends jusqu'à 30 secondes après les tables"
            n212 = Not(x=w414) -> (.not. x?=w415:bool)
            n213 = call "Max-iteration.vi"("i max"=300, "i act"=w418, "Valeur entrante"=w415) -> ("break ?"=w417:bool)
            n214 = Wait Until Next ms Multiple(millisecond multiple=u32 200) -> ()  [unwired: 1 out]
          }
          n215 = while {
            tunnel: [w413] -> w315
            tunnel: w299 -> [w412]
            tunnel: [w405] -> w314
            tunnel: [w404] -> w310
            tunnel: w298 -> [w403]
            tunnel: w307 -> [w402]
            tunnel: [w402] -> w306
            i -> [w408]
            stop <- w406 stop-if-true
            n216 = call "EXCOM-26.vi"("VRN IN"=w412, "Bool Refnum"=w402, "Error IN"=w403) -> ("STATL"=w410:bool[], "VRN OUT"=w413:refnum<visa-resource-name>, "Error OUT"=w404:errorcluster)  [unwired: 6 in, 4 out]
            n217 = Wait Until Next ms Multiple(millisecond multiple=u32 100 ("n millisecondes")) -> ()  [unwired: 1 out]
            n218 = Index Array(array=w410, index=7 ("Index")) -> (element=w405:bool)
            n219 = call "Max-iteration.vi"("i max"=30, "i act"=w408, "Valeur entrante"=w405) -> ("break ?"=w406:bool)
          }
          n220 = case shown="Vrai" w314 {
            selector: w314 -> [w381 _]
            tunnel: w315 -> [w380 w388]
            tunnel: [w381 w387] -> w313
            tunnel: w310 -> [w379 w386]
            tunnel: [w380 w385] -> w309
            tunnel: [w379 w384] -> w308
            tunnel: w306 -> [w378 w383]
            tunnel: [w378 w382] -> w305
            frame False {
            }
            frame True {
              n221 = while {
                tunnel: w388 -> [w398]
                tunnel: [w393] -> w387
                tunnel: w386 -> [w392]
                tunnel: [w391] -> w384
                tunnel: [w390] -> w385
                tunnel: w383 -> [w389]
                tunnel: [w389] -> w382
                i -> [w395]
                stop <- w394 stop-if-true
                n222 = call "EXCOM-26.vi"("VRN IN"=w398, "Bool Refnum"=w389, "Error IN"=w392) -> ("STATL"=w399:bool[], "VRN OUT"=w390:refnum<visa-resource-name>, "Error OUT"=w391:errorcluster)  [unwired: 6 in, 4 out]
                n223 = Index Array(array=w399, index=7 ("Index")) -> (element=w400:bool)
                n224 = Wait Until Next ms Multiple(millisecond multiple=u32 100 ("n millisecondes")) -> ()  [unwired: 1 out]
                n225 = Not(x=w400) -> (.not. x?=w393:bool)
                n226 = call "Max-iteration.vi"("i max"=300, "i act"=w395, "Valeur entrante"=w393) -> ("break ?"=w394:bool)
              }
            }
          }
          n227 = local read "Error Comment"() -> (w302:string)
          n228 = Not(x=w313) -> (.not. x?=w311:bool)
          n229 = Or(x=w311, y=w304) -> (x .or. y?=w312:bool)
          n230 = case shown="Vrai" w312 {
            tunnel: w311 -> [_ w338]
            tunnel: w304 -> [w316 w334]
            tunnel: w309 -> [w319 w332]
            tunnel: w308 -> [w318 w331]
            tunnel: [w319 w329] -> w301
            tunnel: [w318 w330] -> w300
            tunnel: w305 -> [_ w328]
            tunnel: [w317 w326] -> w303
            tunnel: w302 -> [w317 w325]
            frame False {
              # "Enlever dans BonOMM.vi\nvestige de l'interaction avec MaximDL"
              n231 = disable-structure shown="Disabled" {
                disable-tunnel: w316 -> [w320 _]
                frame Disabled {
                  n232 = local read "Guiding"() -> (w323:bool)
                  n233 = local read "Undo startguide"() -> (w322:bool)
                  n234 = Compound Arithmetic op=AND(invert w320, w323, invert w322) -> (w321:bool)
                  n235 = case shown="Vrai" w321 {
                    selector: w321 -> [_ w324]
                    frame False {
                    }
                    frame True {
                      n236 = global write "Globals.vi" "StartGuide"(w324) -> ()
                    }
                  }
                }
                frame Enabled {
                }
              }
            }
            frame True {
              n237 = local read "Error code"() -> (w337:u8)
              n238 = case shown="Vrai" w338 {
                tunnel: [w350 w361] -> w336
                tunnel: w337 -> [w350 w365]
                tunnel: w332 -> [w349 w360]
                tunnel: w331 -> [w348 w359]
                tunnel: [w348 w356] -> w330
                tunnel: [w349 w357] -> w329
                tunnel: w328 -> [_ w354]
                tunnel: [w347 w352] -> w327
                tunnel: w325 -> [w347 w351]
                frame False {
                }
                frame True {
                  n239 = call "EXCOM-CMD.vi"("VRN IN"=w360, "Bool Refnum"=w354, "Commande #"=13 ("NombredArguments"), "Error IN"=w359) -> ("VRN OUT"=w358:refnum<visa-resource-name>, "OK Done"=w363:bool, "Error OUT"=w355:errorcluster)  [unwired: 9 in]
                  n240 = Or(x=w365, y=u8 4) -> (x .or. y?=w362:u8)
                  n241 = case shown="Faux" w363 {
                    tunnel: w362 -> [w370 w377]
                    tunnel: [w369 w377] -> w361
                    tunnel: [w368 w376] -> w357
                    tunnel: w358 -> [w368 w376]
                    tunnel: [w367 w375] -> w356
                    tunnel: w355 -> [w367 w375]
                    frame False {
                      # "Ajoute le bit d'urgence !!!"
                      n242 = local read "Warning code"() -> (w372:u8)
                      n243 = Or(x=w372, y=u8 128) -> (x .or. y?=w373:u8)
                      n244 = Or(x=w370, y=u8 64) -> (x .or. y?=w369:u8)
                      n245 = local write "Warning code"(w373) -> ()
                    }
                    frame True {
                    }
                  }
                  n246 = Concatenate Strings(w351, "Attention, le télescope ne s'est pas arrêter !!!\n") -> (w352:string)
                }
              }
              n247 = case shown="Faux" w334 {
                tunnel: [w340 w345] -> w335
                tunnel: w336 -> [w340 w344]
                tunnel: w327 -> [w339 w342]
                tunnel: [w339 w341] -> w326
                frame False {
                }
                frame True {
                  n248 = Or(x=w344, y=u8 8) -> (x .or. y?=w345:u8)
                  n249 = Concatenate Strings(w342, "Attention, les tables n'ont pas atteintes leur position !!!\n") -> (w341:string)
                }
              }
              n250 = local write "Undo offset"(TRUE ("Undo offset")) -> ()
              n251 = local write "Error code"(w335) -> ()
            }
          }
          n252 = local write "TCS Error"(w300) -> ()
          n253 = local write "TCS VRN"(w301) -> ()
          n254 = local write "Error Comment"(w303) -> ()
        }
        frame True {
        }
      }
    }
    frame #9 {
      n255 = while {
        tunnel: [w430] -> w420
        i -> [w434]
        stop <- w433 stop-if-true
        n256 = local read "TabMove"() -> (w436:refnum<vi>)
        n257 = property class="Bool (strict)"(reference=w436) -> ("Value"=w435:bool)  [unwired: 1 in, 2 out]
        n258 = Wait (ms)(milliseconds to wait=u32 100) -> ()  [unwired: 1 out]
        n259 = Not(x=w435) -> (.not. x?=w430:bool)
        n260 = call "Max-iteration.vi"("i max"=300, "i act"=w434, "Valeur entrante"=w430) -> ("break ?"=w433:bool)
      }
      n261 = case shown="Faux" w420 {
        frame False {
          n262 = local read "Error Comment"() -> (w423:string)
          n263 = local read "Warning code"() -> (w427:u8)
          n264 = local read "Error code"() -> (w426:u8)
          n265 = Concatenate Strings(w423, "Les tables ne semblent pas s'être arrêtées") -> (w422:string)
          n266 = Or(x=w426, y=u8 8) -> (x .or. y?=w425:u8)
          n267 = Or(x=w427, y=u8 8) -> (x .or. y?=w428:u8)
          n268 = local write "Warning code"(w428) -> ()
          n269 = local write "Error code"(w425) -> ()
          n270 = local write "Error Comment"(w422) -> ()
        }
        frame True {
        }
      }
    }
    frame #10 {
      # "Éventuellement, mettre un nombre d'itération de caméra au lieu d'un délai ...\nquoique, il faudrait voir comment tout ça s'harmonise avec un délai PCE ?!?"
      n271 = local read "Guiding"() -> (w439:bool)
      n272 = local read "Undo offset"() -> (w441:bool)
      n273 = Not(x=w441) -> (.not. x?=w440:bool)
      n274 = And(x=w440, y=w439) -> (x .and. y?=w438:bool)
      n275 = case shown="Vrai" w438 {
        tunnel: [TRUE w453] -> w437
        frame False {
        }
        frame True {
          # "Attends 30 secondes que le guidage reparte ..."
          n276 = flat-sequence {
            tunnel: [w464] -> w452
            tunnel: [w474] -> w453
            tunnel: w452 -> [w473]
            frame #0 {
              # "Change le mode ?"
              n277 = local read "Mode"() -> (w455:refnum<vi>)
              n278 = local read "GuiderMode"() -> (w454:u16)
              n279 = property class="MDér (strict)"(reference=w455, "Value"=w454) -> ()  [unwired: 1 in, 2 out]
            }
            frame #1 {
              n280 = local read "StartServo"() -> (w457:refnum<vi>)
              n281 = property class="Bool (strict)"(reference=w457, "Val(Sgnl)"=TRUE ("Value")) -> ()  [unwired: 1 in, 2 out]
            }
            frame #2 {
              n282 = while {
                tunnel: [w458] -> _
                i -> [w462]
                stop <- w460 stop-if-true
                n283 = local read "Servo"() -> (w459:refnum<vi>)
                n284 = Wait (ms)(milliseconds to wait=u32 100) -> ()  [unwired: 1 out]
                n285 = property class="Bool (strict)"(reference=w459) -> ("Value"=w458:bool)  [unwired: 1 in, 2 out]
                n286 = call "Max-iteration.vi"("i max"=300, "i act"=w462, "Valeur entrante"=w458) -> ("break ?"=w460:bool)
              }
            }
            frame #3 {
              n287 = while {
                tunnel: [w467] -> w464
                i -> [w468]
                stop <- w465 stop-if-true
                n288 = local read "SNR"() -> (w472:refnum<vi>)
                n289 = property class="NumNb (strict)"(reference=w472) -> ("Value"=w471:dbl)  [unwired: 1 in, 2 out]
                n290 = Wait Until Next ms Multiple(millisecond multiple=u32 100 ("n millisecondes")) -> ()  [unwired: 1 out]
                n291 = Greater Or Equal?(x=w471, y=5.0) -> (x >= y?=w467:bool)
                n292 = call "Max-iteration.vi"("i max"=100, "i act"=w468, "Valeur entrante"=w467) -> ("break ?"=w465:bool)
              }
            }
            frame #4 {
              n293 = case shown="Vrai" w473 {
                tunnel: [TRUE w485] -> w474
                frame False {
                  n294 = local read "Error Comment"() -> (w481:string)
                  n295 = local read "Warning code"() -> (w477:u8)
                  n296 = local read "Error code"() -> (w478:u8)
                  n297 = Or(x=w478, y=u8 16) -> (x .or. y?=w479:u8)
                  n298 = Or(x=w477, y=u8 16) -> (x .or. y?=w476:u8)
                  n299 = Concatenate Strings(w481, "Il ne semble plus y avoir d'étoile dans la ROI.") -> (w482:string)
                  n300 = local write "Warning code"(w476) -> ()
                  n301 = local write "Error code"(w479) -> ()
                  n302 = local write "Error Comment"(w482) -> ()
                }
                frame True {
                  n303 = while {
                    tunnel: [w491] -> w485
                    i -> [w494]
                    stop <- w493 stop-if-true
                    n304 = local read "Diff Y"() -> (w489:refnum<vi>)
                    n305 = local read "Diff X"() -> (w490:refnum<vi>)
                    n306 = property class="NumNb (strict)"(reference=w490) -> ("Value"=w487:dbl)  [unwired: 1 in, 2 out]
                    "Value X" <- w487
                    n307 = property class="NumNb (strict)"(reference=w489) -> ("Value"=w488:dbl)  [unwired: 1 in, 2 out]
                    "Value Y" <- w488
                    n308 = Wait Until Next ms Multiple(millisecond multiple=u32 100 ("n millisecondes")) -> ()  [unwired: 1 out]
                    n309 = Not Equal To 0?(x=w488) -> (x != 0?=w497:bool)
                    n310 = Not Equal To 0?(x=w487) -> (x != 0?=w496:bool)
                    n311 = call-poly "Pytagore.vi"("D2"=w488, "D1"=w487) -> ("DT"=w499:dbl)
                    n312 = Less?(x=w499, y="OffsetAccuracy (pixels)") -> (x < y?=w495:bool)
                    n313 = Compound Arithmetic op=AND(w495, w496, w497) -> (w491:bool)
                    n314 = call "Max-iteration.vi"("i max"=300, "i act"=w494, "Valeur entrante"=w491) -> ("break ?"=w493:bool)
                  }
                }
              }
            }
          }
        }
      }
      n315 = case shown="Faux" w437 {
        frame False {
          n316 = local read "Error Comment"() -> (w444:string)
          n317 = local read "Warning code"() -> (w448:u8)
          n318 = local read "Error code"() -> (w447:u8)
          n319 = Concatenate Strings(w444, "L'étoile ne s'est pas recentrée, peut-être\npouvez-vous simplement attendre ?\n") -> (w443:string)
          n320 = Or(x=w447, y=u8 16) -> (x .or. y?=w446:u8)
          n321 = Or(x=w448, y=u8 16) -> (x .or. y?=w449:u8)
          n322 = local write "Warning code"(w449) -> ()
          n323 = local write "Error code"(w446) -> ()
          n324 = local write "Error Comment"(w443) -> ()
        }
        frame True {
        }
      }
    }
    frame #11 {
      # "Fermeture"
    }
  }
